vi "MultiChannelType_1D-Array-CDB.vi"(9 "error in":errorcluster, 11 "Array in":cdb[](array[numeric])) -> (1 "error out":errorcluster, 2 "MultiChannelType":cdb, 3 "Array out":cdb[](array[numeric]))   [LabVIEW 2020, in "OpenLvVision_OpenCv.lvlib"]
uses:
  OpenLvVision_OpenCv.lvlib
  <vilib>/Utility/error.llb/Error Cluster From Error Code.vi
  <vilib>/ErrorRing/Error Ring.xnode
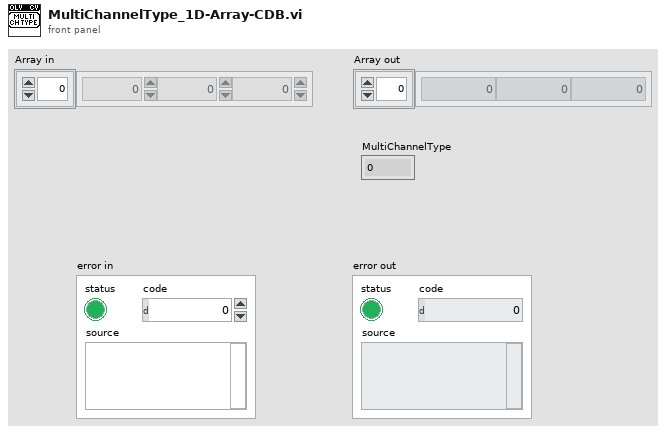
[diagram p1: front panel]
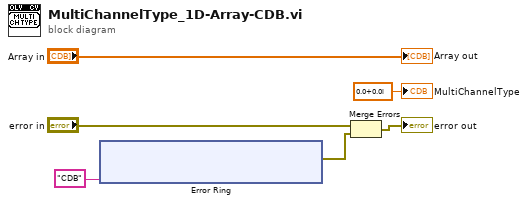
[diagram p0: block diagram]
diagram:
  n1 = xnode "Error Ring"("parameter 0"="CDB") -> ("error out"=w1:errorcluster)
  n2 = Merge Errors("error in", w1) -> (→"error out":errorcluster)
  "Array out" <- "Array in"
  "MultiChannelType" <- csg 0.0+0.0i
